vi "ReadConfiguration.vi"() -> ()   [LabVIEW 2015]
uses:
  <vilib>/Utility/config.llb/Read Key (String).vi
  <vilib>/Utility/config.llb/NI_LVConfig.lvlib
panel:
  out "Array":string[][](array[string])
  out "error out":errorcluster
  in  "error in":errorcluster
  in  "File Path Control":path
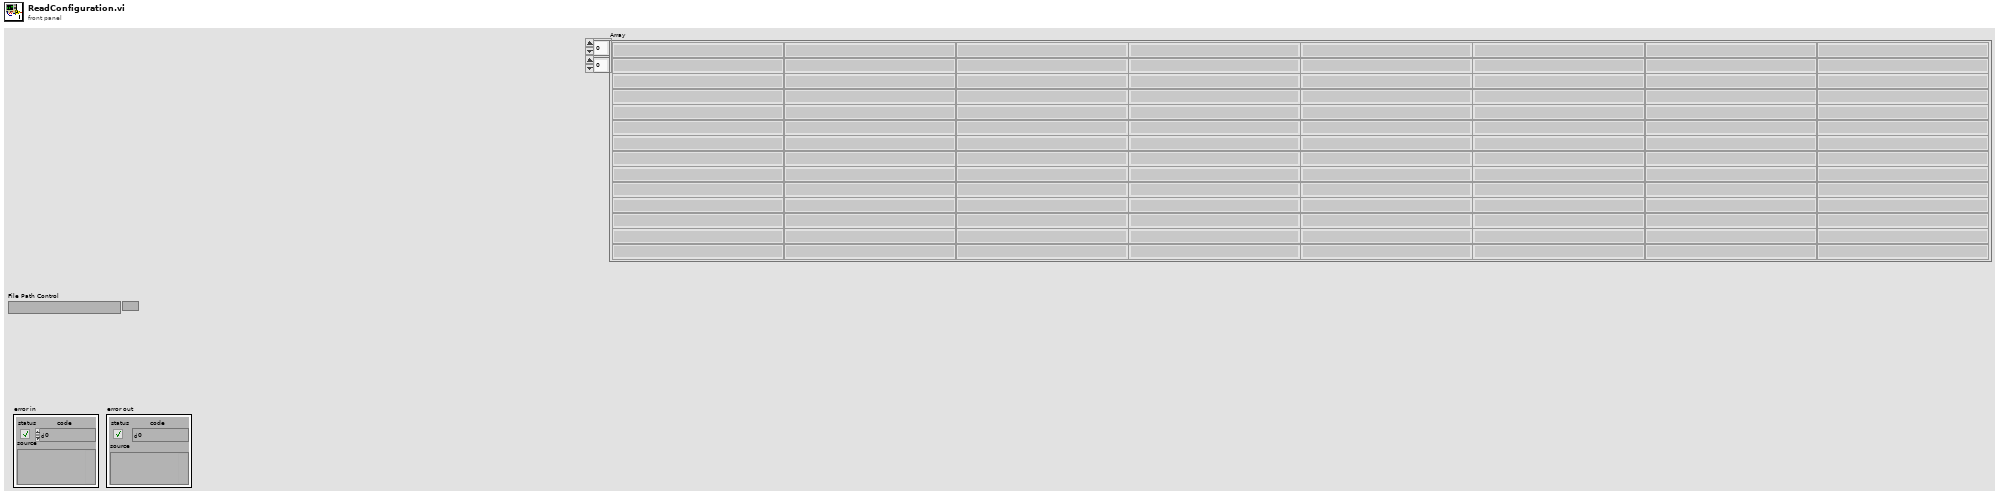
[diagram p1: front panel]
types:
  T1 = typedef "NI_LVConfig.lvlib/Config Data RefNum.ctl" = refnum<k1>
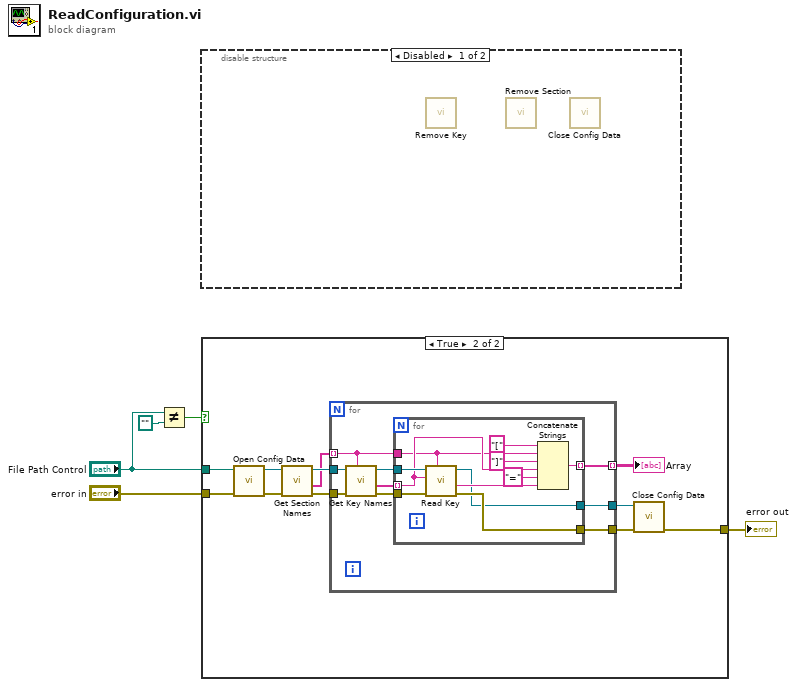
[diagram p0: block diagram]
diagram:
  n1 = Not Equal?(x="File Path Control", y=path "") -> (x != y?=w3:bool)
  n2 = disable-structure shown="Disabled" {
    frame Disabled {
      n3 = call <vilib>:"Remove Key.vi"() -> ()  [unwired: 9 in, 3 out]
      n4 = call <vilib>:"Remove Section.vi"() -> ()  [unwired: 9 in, 3 out]
      n5 = call <vilib>:"Close Config Data.vi"() -> ()  [unwired: 10 in, 2 out]
    }
    frame Enabled {
    }
  }
  n6 = case shown="True" w3 {
    tunnel: [w6 w16] -> w5
    tunnel: "File Path Control" -> [_ w17]
    tunnel: "error in" -> [w6 w15]
    frame False {
    }
    frame True {
      n7 = call <vilib>:"Open Config Data.vi"("error in (no error)"=w15, "configuration file path"=w17) -> ("error out"=w14:errorcluster, "refnum"=w13:T1)  [unwired: 7 in, 1 out]
      n8 = call <vilib>:"Get Section Names.vi"("error in (no error)"=w14, "refnum"=w13) -> ("error out"=w11:errorcluster, "section names"=w10:string[], "refnum out"=w12:T1)  [unwired: 7 in]
      n9 = for {
        tunnel: w12 -> [w26]
        tunnel: w11 -> [w25]
        tunnel: w10 -> [w22] mode=indexing
        tunnel: [w20] -> w7
        tunnel: [w19] -> w9 mode=indexing
        tunnel: [w18] -> w8
        n10 = call <vilib>:"Get Key Names.vi"("section"=w22, "error in (no error)"=w25, "refnum"=w26) -> ("error out"=w23:errorcluster, "key names"=w21:string[], "refnum out"=w24:T1)  [unwired: 5 in, 1 out]
        n11 = for {
          tunnel: w24 -> [w37]
          tunnel: w23 -> [w36]
          tunnel: w22 -> [w29]
          tunnel: w21 -> [w34] mode=indexing
          tunnel: [w35] -> w20
          tunnel: [w31] -> w19 mode=indexing
          tunnel: [w28] -> w18
          n12 = call-poly <vilib>:"Read Key.vi"("section"=w29, "error in (no error)"=w36, "key"=w34, "refnum"=w37) -> ("error out"=w35:errorcluster, "value"=w32:string, "refnum out"=w28:T1)  [unwired: 4 in, 1 out]
          n13 = Concatenate Strings("[" ("string"), w29, "]" ("string"), w34, "=" ("string"), w32) -> (w31:string)
        }
      }
      "Array" <- w9
      n14 = call <vilib>:"Close Config Data.vi"("error in (no error)"=w7, "refnum"=w8) -> ("error out"=w16:errorcluster)  [unwired: 8 in, 1 out]
    }
  }
  "error out" <- w5
